vi "File_SetupTDMS.vi"(8 "error in (no error)":errorcluster, 11 "File in":refnum<class "File.lvclass">) -> (0 "error out":errorcluster, 3 "File out":refnum<class "File.lvclass">)   [LabVIEW 2023, in "File.lvclass"]
doc: "Creates the TDMS file as defined in the class."
uses:
  File.lvclass
  File.lvclass/File.ctl
  Group/Group.lvclass
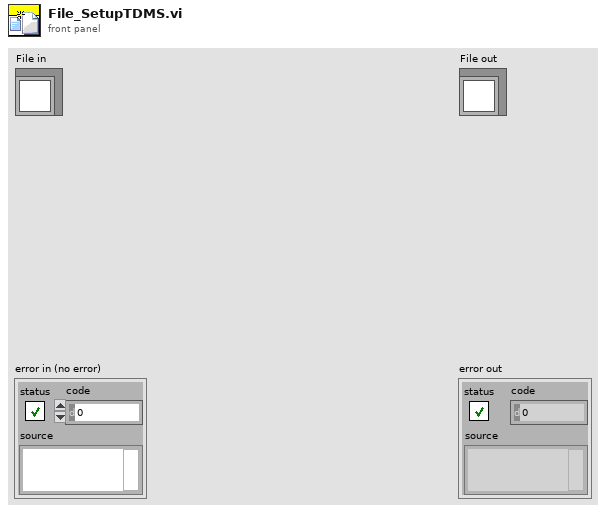
[diagram p1: front panel]
types:
  T1 = enum16{"open", "open or create", "create or replace", "create", "open (read-only)"}
  T2 = typedef "Meta Data.ctl" = cluster{"Key":string, "Value":string}
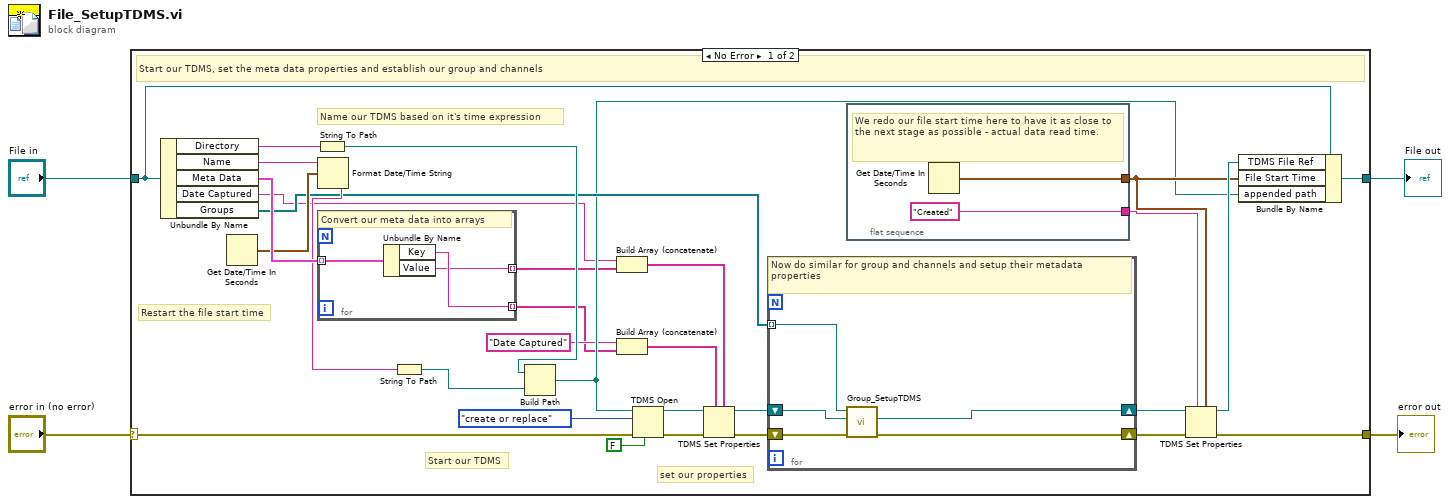
[diagram p0: block diagram]
diagram:
  n1 = case shown="No Error" "error in (no error)" {
    selector: "error in (no error)" -> [w23 w46]
    tunnel: [w20 w46] -> w3
    tunnel: [w15 w45] -> w1
    tunnel: "File in" -> [w18 w45]
    frame No Error {
      # "set our properties"
      # "Name our TDMS based on it's time expression"
      # "Start our TDMS"
      # "Restart the file start time"
      # "Start our TDMS, set the meta data properties and establish our group and channels"
      n2 = Unbundle By Name(w18) -> ("Directory"=w26:string, "Name"=w30:string, "Meta Data"=w32:T2[], "Date Captured"=w9:string, "Groups"=w25:refnum<class "Group.lvclass">[])
      n3 = Get Date/Time In Seconds() -> (seconds since 1Jan1904=w31:timestamp)
      n4 = String To Path(string=w26) -> (path=w29:path)
      n5 = Format Date/Time String(time format string (%c)=w30, seconds (now)=w31) -> (date/time string=w27:string)  [unwired: 1 in]
      n6 = for {
        tunnel: w32 -> [w44] mode=indexing
        tunnel: [w43] -> w11 mode=indexing
        tunnel: [w42] -> w8 mode=indexing
        # "Convert our meta data into arrays"
        n7 = Unbundle By Name(w44) -> ("Key"=w43:string, "Value"=w42:string)
      }
      n8 = String To Path(string=w27) -> (path=w28:path)
      n9 = Build Path(base path=w29, name or relative path=w28) -> (appended path=w14:path)
      n10 = Build Array (concatenate)(w9, w8) -> (w7:string[])
      n11 = Build Array (concatenate)("Date Captured", w11) -> (w10:string[])
      n12 = TDMS Open(6:FALSE ("disable buffering? (T)"), 8:w23, 10:T1."create or replace" ("operation (0:open)"), 11:w14) -> (0:w5:errorcluster, 3:w6:refnum<k34>)  [unwired: 3 in]
      n13 = TDMS Set Properties(5:w7, 7:w10, 8:w5, 11:w6) -> (0:w24:errorcluster, 3:w22:refnum<k34>)  [unwired: 1 in, 3 out]
      n14 = for {
        tunnel: w25 -> [w41] mode=indexing
        shift-right: [w38] -> w21
        shift-left: w24 -> [w39]
        shift-right: [w37] -> w13
        shift-left: w22 -> [w40]
        # "Now do similar for group and channels and setup their metadata properties"
        n15 = call-dynamic "Group_SetupTDMS.vi"("error in (no error)"=w39, "tdms file in"=w40, "Group in"=w41) -> ("error out"=w38:errorcluster, "tdms file out"=w37:refnum<k34>)  [unwired: 6 in, 1 out]
      }
      n16 = flat-sequence {
        tunnel: [w36] -> w16
        tunnel: ["Created" ("Name")] -> w19
        frame #0 {
          # "We redo our file start time here to have it as close to the next stage as possible - actual data read time."
          n17 = Get Date/Time In Seconds() -> (seconds since 1Jan1904=w36:timestamp)
        }
      }
      n18 = TDMS Set Properties(5:w16, 7:w19, 8:w21, 11:w13) -> (0:w20:errorcluster, 3:w17:refnum<k34>)  [unwired: 1 in, 3 out]
      n19 = Bundle By Name(cluster=w18, "TDMS File Ref"=w17, "File Start Time"=w16, "appended path"=w14) -> (w15:refnum<class "File.lvclass">)
    }
    frame Error {
    }
  }
  "error out" <- w3
  "File out" <- w1
